vi "Generate XML String from Report Class.vi"(8 "error in (no error)":errorcluster caption="Fehler (Eingang, kein Fehler)", 10 "Dateipfad (Dialog verwenden)":path, 11 "Daten":T1={"Report.lvclass"=refnum, "Norm"="", "last State"=enum."Initialize", "Norm ID"=0, "parameter"=[], "EMTestCWS500N.lvclass"=refnum, "CEG4500.lvclass"=refnum, "Tektronix RSA5106A.lvclass"=refnum, "erfolgreich"=FALSE, "log"="", "Kommentar"="", "Device Enum"=enum."emTestCWS500N", "Test Enum"=enum."HF-Felder", "debug"=FALSE, "tab"=enum."Hauptmenü"}) -> (0 "Fehler (Ausgang)":errorcluster)   [LabVIEW 2013, in "XML.lvlib"]
doc: "Dieses Vi erstellt aus der Datenstruktur eine Xml-Datei. Wenn die Prüfdaten nicht gespeichtert werden kann der Prüfprozess nicht wieder bearbeitet werden. Die Pdf-Datei ist nicht zum laden dieser Informationen geeignet."
uses:
  lib/XML.lvlib
  Main/controls/Data.ctl
  classes/Datastructure/Report/Report.lvclass
  classes/Devices/emTestCWS500N/EMTestCWS500N.lvclass
  classes/Devices/CEG4500/CEG4500.lvclass
  classes/Devices/Tektronix RSA5106A/Tektronix RSA5106A.lvclass
  Main/controls/State.ctl
  classes/Devices/DeviceInterface/Devices.ctl
  classes/Tests/TestInterface/Tests.ctl
  Tabs.ctl
  classes/Datastructure/Norm/Norm.lvclass
  classes/Datastructure/Setup/Setup.lvclass
  classes/Datastructure/Image/img.lvclass
  classes/Datastructure/Device/Device.lvclass
  classes/Datastructure/Test/Test.lvclass
  <vilib>/xml/Close Reference(Node).vi
  <resource>/objmgr/DOMUserDefRef.rc
  <vilib>/xml/NI_XML.lvlib
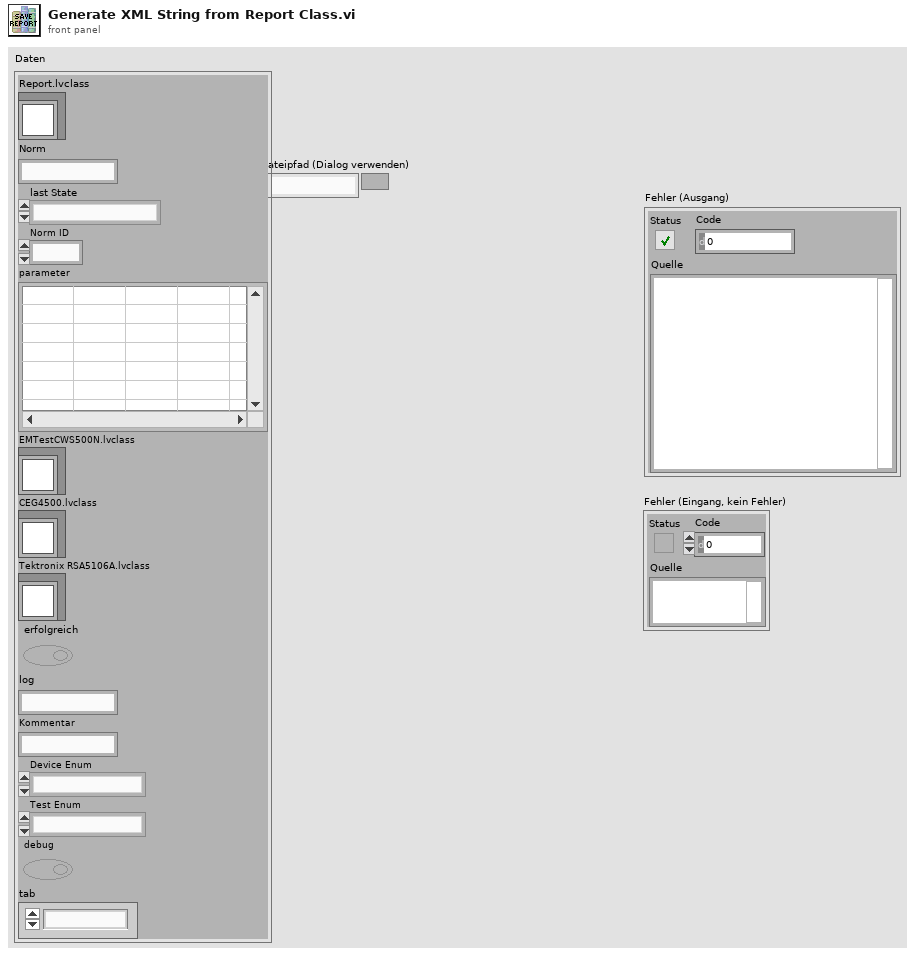
[diagram p1: front panel]
types:
  T1 = typedef "Data.ctl" = cluster{"Report.lvclass":refnum<class "Report.lvclass">, "Norm":string, "last State":T2, "Norm ID":i32, "parameter":string[][], "EMTestCWS500N.lvclass":refnum<class "EMTestCWS500N.lvclass">, "CEG4500.lvclass":refnum<class "CEG4500.lvclass">, "Tektronix RSA5106A.lvclass":refnum<class "Tektronix RSA5106A.lvclass">, "erfolgreich":bool, "log":string, "Kommentar":string, "Device Enum":T3, "Test Enum":T4, "debug":bool, "tab":T5}
  T2 = typedef "State.ctl" = enum16{"create Pdf", "load Report", "save Report", "do Test", "CDN Kalibrierung", "enter Report Parameters", "new Test", "Protokoll", "read Tree", "update Tree", "Fehler", "Initialize", "Wait for Event", "Exit"}
  T3 = typedef "Devices.ctl" = enum16{"unbekannt", "Tektronix RSA5106A", "emTestCWS500N", "CEG-4500"}
  T4 = typedef "Tests.ctl" = enum16{"unbekannt", "Störaussendung", "Burst", "ESD", "Surge", "Spannungseinbruch", "HF-Felder"}
  T5 = typedef "Tabs.ctl" = enum32{"Hauptmenü", "Prüfbericht", "Einstellungen"}
  T6 = enum16{"open", "replace", "create", "open or create", "replace or create", "replace or create with confirmation"}
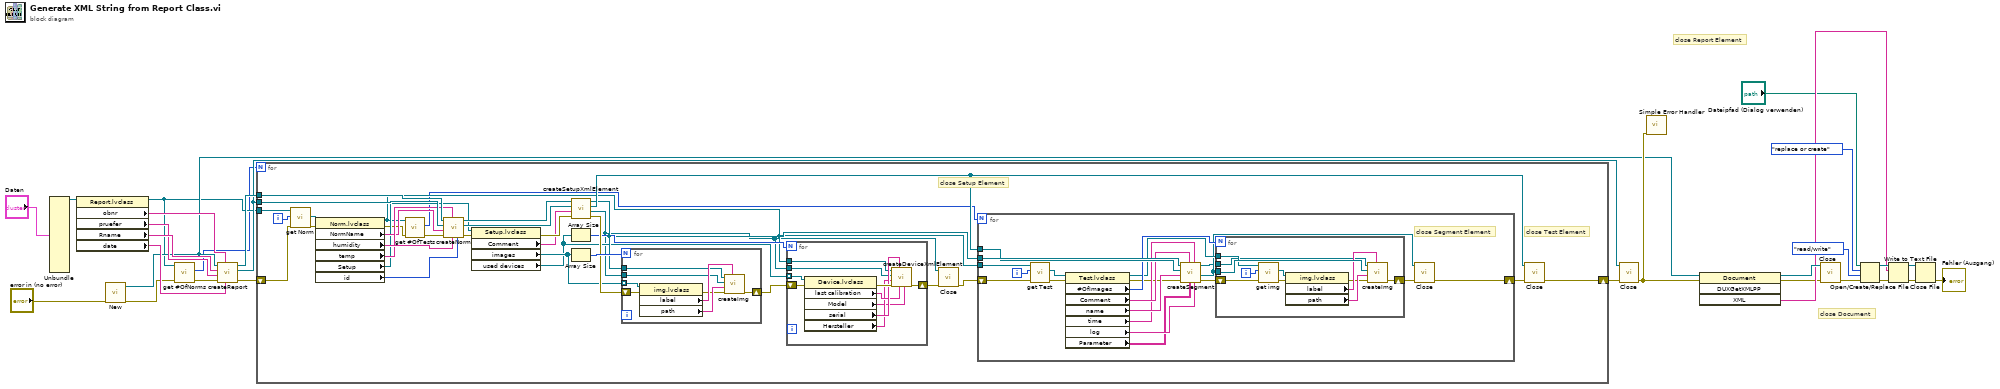
[diagram p0: block diagram]
diagram:
  # "close Document"
  # "close Report Element"
  n1 = Unbundle("Daten") -> ("Report.lvclass"=w19:refnum<class "Report.lvclass">)  [unwired: 14 out]
  n2 = property class="Report.lvclass"(reference=w19) -> (reference out=w5:refnum<class "Report.lvclass">, "obnr"=w16:string, "pruefer"=w17:string, "Rname"=w18:string, "date"=w8:string)  [unwired: 1 in, 1 out]
  n3 = call <vilib>:"New.vi"("error in (no error)"="error in (no error)") -> ("error out"=w3:errorcluster, "DOM document out"=w7:refnum<k20>)  [unwired: 7 out]
  n4 = call-dynamic "get #OfNorms.vi"("error in (no error)"=w3, "Report (Eingang)"=w5) -> ("error out"=w2:errorcluster, "#OfTests"=w4:u32)  [unwired: 7 in, 1 out]
  n5 = call "createReport.vi"("date"=w8, "obrn"=w16, "error in (no error)"=w2, "pruefer"=w17, "Baugruppenname"=w18, "DOM Document"=w7) -> ("error out"=w20:errorcluster, "Report ref"=w6:refnum<k20>, "dup DOM Document"=w21:refnum<k20>)  [unwired: 3 in]
  n6 = for {
    N: w4 -> [_]
    tunnel: w6 -> [w60]
    shift-right: [w63] -> w15
    shift-left: w20 -> [w58]
    tunnel: w5 -> [w59]
    tunnel: w21 -> [w61]
    i -> [w56]
    # "close Test Element"
    # "close Setup Element"
    n7 = call-dynamic "get Norm.vi"("error in (no error)"=w58, "index"=w56, "Report (Eingang)"=w59) -> ("error out"=w55:errorcluster, "Test.lvclass"=w57:refnum<class "Norm.lvclass">)  [unwired: 6 in, 1 out]
    n8 = property class="Norm.lvclass"(reference=w57, error in=w55) -> (reference out=w33:refnum<class "Norm.lvclass">, error out=w31:errorcluster, "NormName"=w52:string, "humidity"=w54:string, "temp"=w53:string, "Setup"=w36:refnum<class "Setup.lvclass">, "id"=w35:i32)
    n9 = call-dynamic "get #OfTests.vi"("error in (no error)"=w31, "Norm (Eingang)"=w33) -> ("error out"=w30:errorcluster, "#OfTests"=w32:u32)  [unwired: 7 in, 1 out]
    n10 = call "createNorm.vi"("id"=w35, "humidity"=w54, "temp"=w53, "error in (no error)"=w30, "TestName"=w52, "report ref"=w60, "DOM document"=w61) -> ("error out"=w37:errorcluster, "test ref"=w50:refnum<k20>, "dup DOM document"=w51:refnum<k20>)  [unwired: 1 in, 1 out]
    n11 = property class="Setup.lvclass"(reference=w36, error in=w37) -> (error out=w41:errorcluster, "Comment"=w40:string, "images"=w39:refnum<class "img.lvclass">[], "used devices"=w38:refnum<class "Device.lvclass">[])  [unwired: 1 out]
    n12 = call "createSetupXmlElement.vi"("error in (no error)"=w41, "Comment"=w40, "Test ref"=w50, "DOM document"=w51) -> ("error out"=w47:errorcluster, "Setup ref"=w34:refnum<k20>, "dup Test ref"=w49:refnum<k20>, "dup DOM document"=w44:refnum<k20>)  [unwired: 4 in]
    n13 = Array Size(array=w38) -> (size(s)=w46:i32)
    n14 = Array Size(array=w39) -> (size(s)=w48:i32)
    n15 = for {
      N: w48 -> [_]
      tunnel: w39 -> [w81] mode=indexing
      tunnel: w34 -> [w74]
      tunnel: w44 -> [w77]
      shift-right: [w75] -> w45
      shift-left: w47 -> [w80]
      n16 = property class="img.lvclass"(reference=w81, error in=w80) -> (error out=w76:errorcluster, "label"=w79:string, "path"=w78:string)  [unwired: 1 out]
      n17 = call "createImg.vi"("label"=w79, "error in (no error)"=w76, "path"=w78, "seg ref"=w74, "DOM document"=w77) -> ("error out"=w75:errorcluster)  [unwired: 4 in, 2 out]
    }
    n18 = for {
      N: w46 -> [_]
      tunnel: w38 -> [w73] mode=indexing
      tunnel: w34 -> [w68]
      tunnel: w44 -> [w67]
      shift-right: [w66] -> w43
      shift-left: w45 -> [w72]
      n19 = property class="Device.lvclass"(reference=w73, error in=w72) -> (error out=w71:errorcluster, "last calibration"=w69:string, "Model"=w64:string, "serial"=w70:string, "Hersteller"=w65:string)  [unwired: 1 out]
      n20 = call "createDeviceXmlElement.vi"("model"=w64, "lastcal"=w69, "serial"=w70, "error in (no error)"=w71, "manu"=w65, "setup ref"=w68, "DOM document"=w67) -> ("error out"=w66:errorcluster)  [unwired: 2 in, 2 out]
    }
    n21 = call-poly <vilib>:"Close.vi"("error in (no error)"=w43, "node"=w34) -> ("error out"=w42:errorcluster)  [unwired: 7 out]
    n22 = for {
      N: w32 -> [_]
      tunnel: w49 -> [w99]
      shift-right: [w101] -> w62
      shift-left: w42 -> [w88]
      tunnel: w33 -> [w96]
      tunnel: w44 -> [w100]
      i -> [w89]
      # "close Segment Element"
      n23 = call-dynamic "get Test.vi"("error in (no error)"=w88, "index"=w89, "Norm (Eingang)"=w96) -> ("error out"=w87:errorcluster, "Test.lvclass"=w95:refnum<class "Test.lvclass">)  [unwired: 6 in, 1 out]
      n24 = property class="Test.lvclass"(reference=w95, error in=w87) -> (reference out=w90:refnum<class "Test.lvclass">, error out=w86:errorcluster, "#OfImages"=w91:u32, "Comment"=w93:string, "name"=w94:string, "time"=w92:string, "log"=w84:string, "Parameter"=w83:string[][])
      n25 = call "createSegment.vi"("log"=w84, "time"=w92, "Parameter"=w83, "Comment"=w93, "error in (no error)"=w86, "SegName"=w94, "test ref"=w99, "DOM document"=w100) -> ("error out"=w98:errorcluster, "seg ref"=w85:refnum<k20>, "dup DOM document"=w82:refnum<k20>)  [unwired: 1 out]
      n26 = for {
        N: w91 -> [_]
        tunnel: w85 -> [w112]
        shift-right: [w103] -> w97
        shift-left: w98 -> [w106]
        tunnel: w90 -> [w111]
        tunnel: w82 -> [w102]
        i -> [w110]
        n27 = call-dynamic "get img.vi"("error in (no error)"=w106, "index"=w110, "Test (Eingang)"=w111) -> ("error out"=w105:errorcluster, "img.lvclass"=w109:refnum<class "img.lvclass">)  [unwired: 6 in, 1 out]
        n28 = property class="img.lvclass"(reference=w109, error in=w105) -> (error out=w104:errorcluster, "label"=w107:string, "path"=w108:string)  [unwired: 1 out]
        n29 = call "createImg.vi"("label"=w107, "error in (no error)"=w104, "path"=w108, "seg ref"=w112, "DOM document"=w102) -> ("error out"=w103:errorcluster)  [unwired: 4 in, 2 out]
      }
      n30 = call-poly <vilib>:"Close.vi"("error in (no error)"=w97, "node"=w85) -> ("error out"=w101:errorcluster)  [unwired: 7 out]
    }
    n31 = call-poly <vilib>:"Close.vi"("error in (no error)"=w62, "node"=w49) -> ("error out"=w63:errorcluster)  [unwired: 7 out]
  }
  n32 = call-poly <vilib>:"Close.vi"("error in (no error)"=w15, "node"=w6) -> ("error out"=w11:errorcluster)  [unwired: 7 out]
  n33 = call <vilib>:"Simple Error Handler.vi"("error in (no error)"=w11) -> ()  [unwired: 4 in, 5 out]
  n34 = invoke class="Document" method="DUXGetXMLPP"(reference=w7, error in=w11) -> (reference out=w29:refnum<k20>, error out=w12:errorcluster, "XML"=w22:string)  [unwired: 2 in, 1 out]
  n35 = call-poly <vilib>:"Close.vi"("error in (no error)"=w12, "node"=w29) -> ("error out"=w9:errorcluster)  [unwired: 7 out]
  n36 = Open/Create/Replace File(file path (use dialog)="Dateipfad (Dialog verwenden)", error in=w9, operation (0:open)=T6."replace or create" ("Operation (0:Öffnen)"), access (0:read/write)=enum16{"read/write", "read-only", "write-only"}."read/write" ("Zugriff (0:Lesen/Schreiben)")) -> (refnum out=w23:refnum<file>, error out=w24:errorcluster)  [unwired: 2 in, 1 out]
  n37 = Write to Text File(file (use dialog)=w23, text=w22, error in=w24) -> (refnum out=w28:refnum<file>, error out=w27:errorcluster)  [unwired: 1 in, 1 out]
  n38 = Close File(refnum=w28, error in=w27) -> (error out=→"Fehler (Ausgang)":errorcluster)  [unwired: 1 out]
